vi "Load Analysis Data.vi"(1 "Load Path":path) -> (0 "Loaded Entry":T1)   [LabVIEW 2013]
uses:
  <vilib>/xml/Load XML File.vi
  <vilib>/xml/NI_XML.lvlib
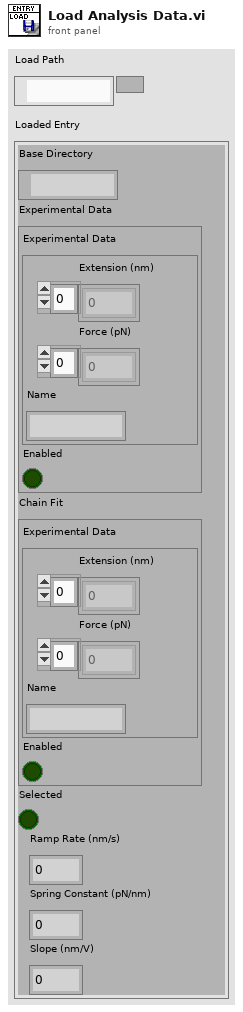
[diagram p1: front panel]
types:
  T1 = cluster{"Base Directory":path, "Experimental Data":cluster{"Experimental Data":cluster{"Extension (nm)":dbl[], "Force (pN)":dbl[], "Name":string}, "Enabled":bool}, "Chain Fit":cluster{"Experimental Data":cluster{"Extension (nm)":dbl[], "Force (pN)":dbl[], "Name":string}, "Enabled":bool}, "Selected":bool, "Ramp Rate (nm/s)":dbl, "Spring Constant (pN/nm)":dbl, "Slope (nm/V)":dbl}
  T2 = typedef "Experiment Data.ctl" = cluster{"Force Data":dbl[], "Signal Strength Data":dbl[], "X Position Data":dbl[], "Y Position Data":dbl[], "Z Position Data":dbl[], "Ramp Rate":dbl, "Z Scan Size":dbl, "Slope":dbl, "Spring Constant":dbl, "Version":string}
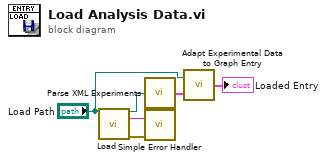
[diagram p0: block diagram]
diagram:
  n1 = call-poly <vilib>:"Load.vi"("path to XML document"="Load Path") -> ("DOM document out"=w6:refnum<k20>, "parse errors"=w4:string, "error out"=w5:errorcluster)  [unwired: 12 in]
  n2 = call "Parse XML Experiments.vi"("DOM"=w6) -> ("Experiment Data"=w3:T2)
  n3 = call <vilib>:"Simple Error Handler.vi"("error source (\" \")"=w4, "error in (no error)"=w5) -> ()  [unwired: 3 in, 5 out]
  n4 = call "Adapt Experimental Data to Graph Entry.vi"("Experiment Data"=w3, "Load Path"="Load Path") -> ("Populated Entry"=→"Loaded Entry":T1)
